vi "GlobalData.vi"() -> ()   [LabVIEW 2017]
uses:
  Controls/ShiftRegisterCluster.ctl
panel:
  in  "Data Cluster":T1
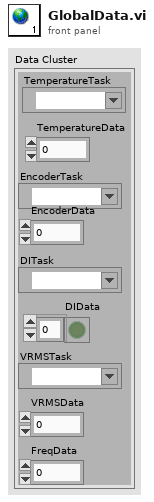
[diagram p1: front panel]
types:
  T1 = typedef "ShiftRegisterCluster.ctl" = cluster{"TemperatureTask":refnum<k21>, "TemperatureData":dbl, "EncoderTask":refnum<k21>, "EncoderData":dbl, "DITask":refnum<k21>, "DIData":bool[], "VRMSTask":refnum<k21>, "VRMSData":dbl, "FreqData":dbl}
diagram:
